vi "write.vi"() -> ()   [LabVIEW 2016]
uses:
  <vilib>/Instr/_visa.llb/VISA Configure Serial Port (Serial Instr).vi
panel:
  in  "Numeric":dbl
  out "Red":bool
  out "yellow":bool
  out "Unit":string
  out "Unit":string
  out "Battery status":bool
  out "Gauge battery Voltage":dbl
  in  "Enable light control":bool
  in  "voltage read length":u32
  out "Voltage feedback":string
  in  "Read":bool
  in  "Cancel Zero reading":bool
  in  "Zero Reading":bool
  in  "Gauge light":bool
  out "Helium underpressure":bool
  out "Numeric 2":dbl
  in  "Set Relay voltage":dbl(slide)=9.0 scale=0.0..10.0
  out "Compressor Status":bool
  in  "Pressure Lower Limit":dbl=0.1
  out "Helium Overpressure":bool
  in  "Pressure Upper Limit":dbl=2.8
  in  "Reading 2":string(combo)="255:R:OTEMP"
  out "Monitor 2":dbl(graph)
  out "Temperature":dbl=23.05
  in  "monitor 2 read length":u32=25
  out "monitor 2 feedback":string
  in  "Reading 1":string(combo)="255:R:MRMD"
  in  "Abort monitoring":bool
  out "Puressure":dbl=0.009
  in  "monitor 1 read length":u32=25
  out "Monitor 1":dbl(graph)
  out "Monitor 1 feedback":string
  # "Gauge Operation"
  # "Relay Configuration"
  # "Serial Port I/O control"
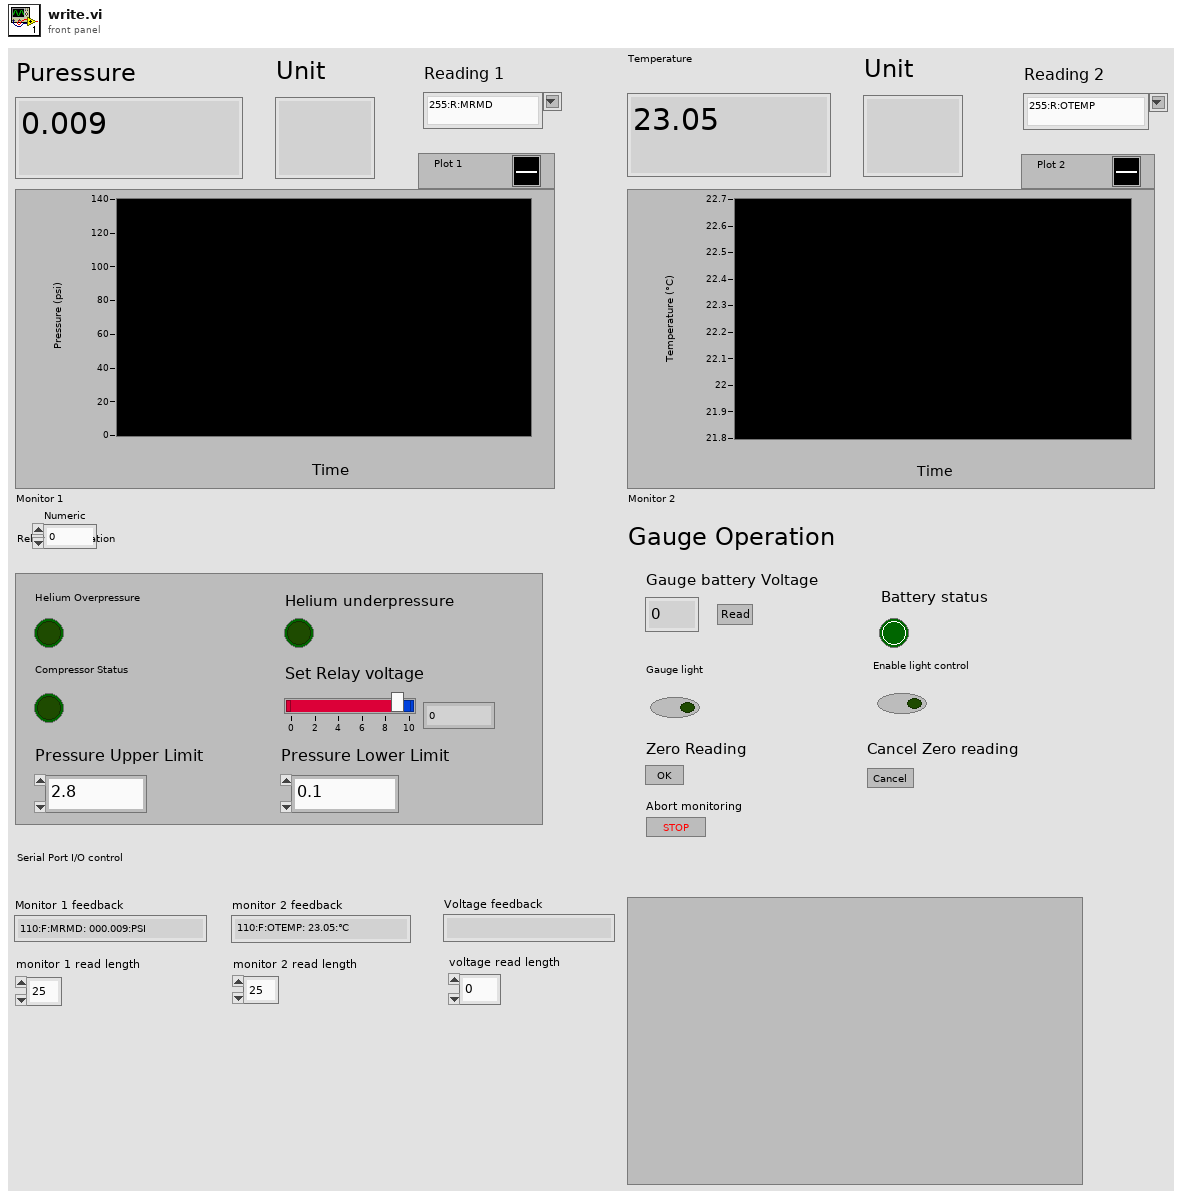
[diagram p1: front panel]
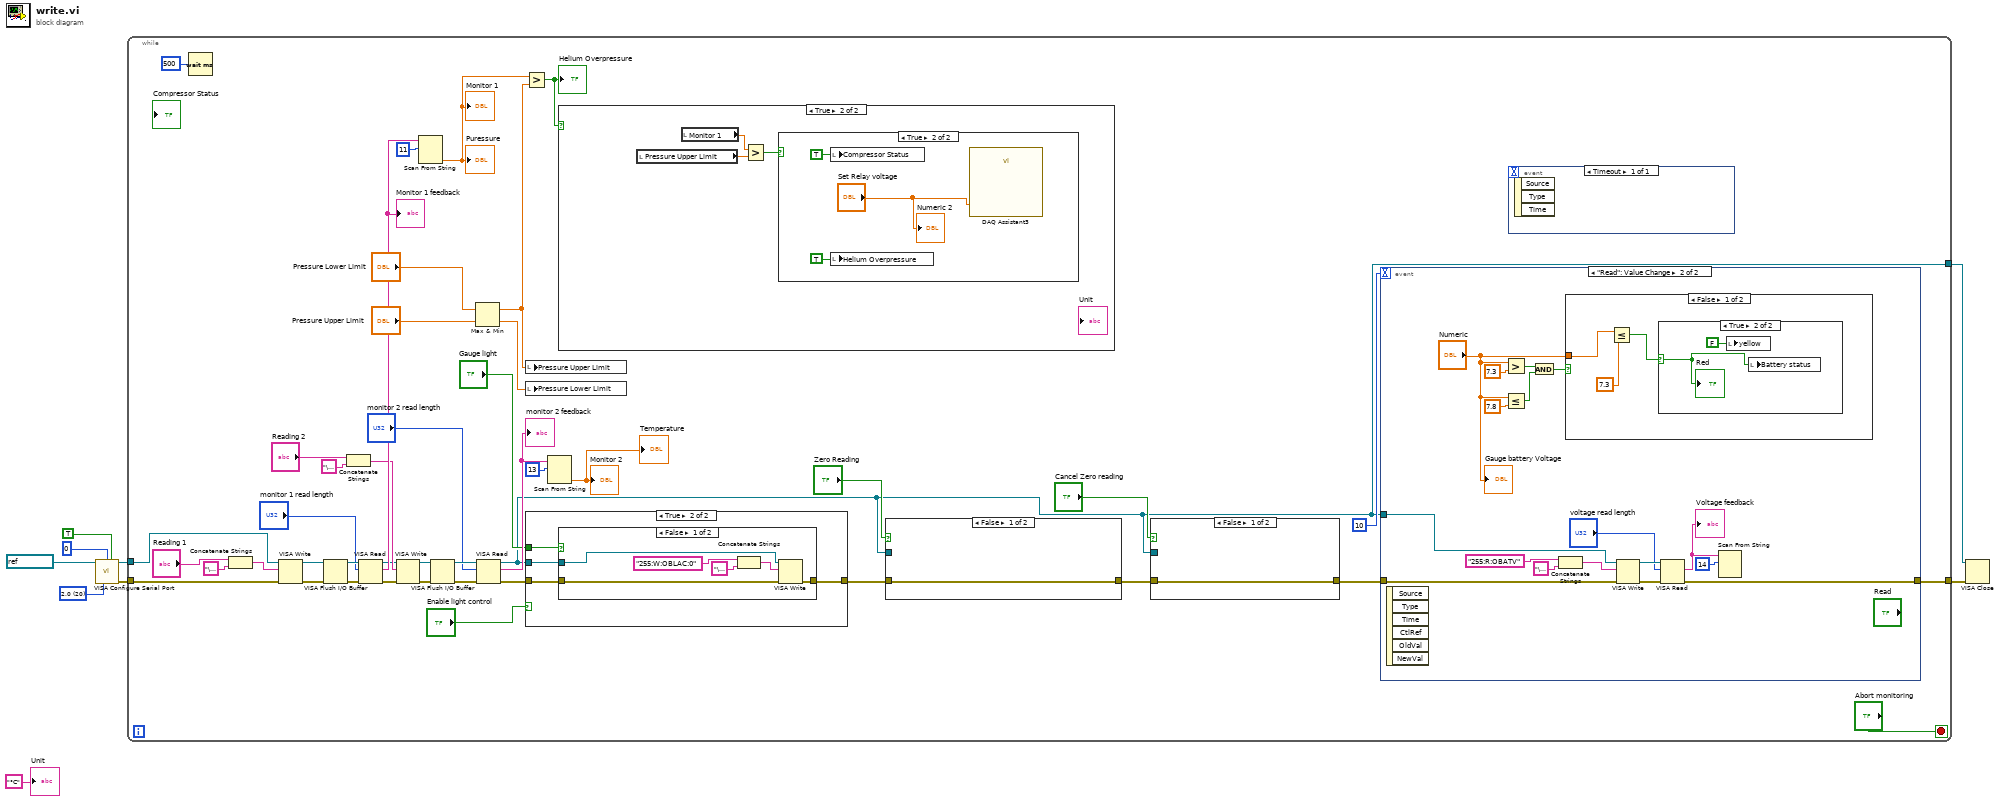
[diagram p0: block diagram]
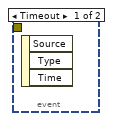
[diagram p2: hidden frame]
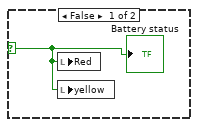
[diagram p3: hidden frame]
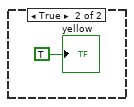
[diagram p4: hidden frame]
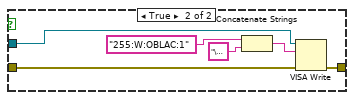
[diagram p6: hidden frame]
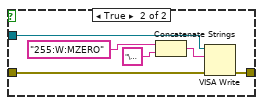
[diagram p7: hidden frame]
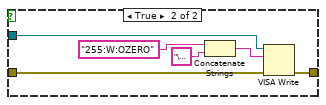
[diagram p8: hidden frame]
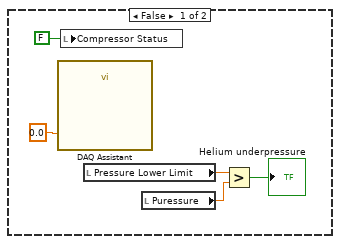
[diagram p9: hidden frame]
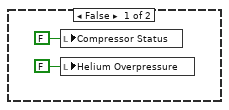
[diagram p10: hidden frame]
diagram:
  w6 = u16 20 items=["1.0"=10, "1.5"=15, "2.0"=20] ("stop bits (10: 1 bit)")
  n1 = call-poly "VISA Configure Serial Port"("VISA resource name"=refnum<visa-resource-name> "COM2", "termination char\n(0xA = '\\n' = LF)"=u8 0 ("termination char\n(0xA = '\\n' = LF)"), "Enable Termination\nChar (T)"=TRUE ("Enable Termination\nChar (T)"), "stop bits (10: 1 bit)"=w6) -> ("VISA resource name out"=w4:refnum<visa-resource-name>, "error out"=w5:errorcluster)  [unwired: 10 in]
  n2 = while {
    tunnel: [w12] -> w3
    tunnel: w5 -> [w45]
    tunnel: w4 -> [w24]
    tunnel: [w10] -> w2
    stop <- "Abort monitoring" stop-if-true
    n3 = Wait (ms)(milliseconds to wait=u32 500) -> ()  [unwired: 1 out]
    n4 = Concatenate Strings("Reading 1", "\u0000") -> (w53:string)
    n5 = VISA Write(VISA resource name=w24, write buffer=w53, error in (no error)=w45) -> (VISA resource name out=w49:refnum<visa-resource-name>, error out=w51:errorcluster)  [unwired: 1 out]
    n6 = VISA Flush I/O Buffer(VISA resource name=w49, error in (no error)=w51) -> (VISA resource name out=w50:refnum<visa-resource-name>, error out=w44:errorcluster)  [unwired: 1 in]
    n7 = Concatenate Strings("Reading 2", "\u0000") -> (w40:string)
    n8 = VISA Read(VISA resource name=w50, byte count="monitor 1 read length", error in (no error)=w44) -> (VISA resource name out=w30:refnum<visa-resource-name>, read buffer=w47:string, error out=w29:errorcluster)  [unwired: 1 out]
    "Monitor 1 feedback" <- w47
    n9 = VISA Write(VISA resource name=w30, write buffer=w40, error in (no error)=w29) -> (VISA resource name out=w36:refnum<visa-resource-name>, error out=w38:errorcluster)  [unwired: 1 out]
    n10 = Scan From String(input string=w47, initial scan location=u32 11) -> (output 1=w21:dbl)  [unwired: 3 in, 3 out]
    "Puressure" <- w21
    "Monitor 1" <- w21
    n11 = VISA Flush I/O Buffer(VISA resource name=w36, error in (no error)=w38) -> (VISA resource name out=w37:refnum<visa-resource-name>, error out=w32:errorcluster)  [unwired: 1 in]
    n12 = Max & Min(x="Pressure Lower Limit", y="Pressure Upper Limit") -> (max(x,y)=w26:dbl, min(x,y)=w25:dbl)
    n13 = VISA Read(VISA resource name=w37, byte count="monitor 2 read length", error in (no error)=w32) -> (VISA resource name out=w12:refnum<visa-resource-name>, read buffer=w34:string, error out=w18:errorcluster)  [unwired: 1 out]
    "monitor 2 feedback" <- w34
    n14 = Greater?(x=w21, y=w26) -> (0:w22:bool)
    "Helium Overpressure" <- w22
    n15 = local write "Pressure Upper Limit"(w26) -> ()
    n16 = local write "Pressure Lower Limit"(w25) -> ()
    n17 = case shown="True" "Enable light control" {
      tunnel: "Gauge light" -> [_ w82]
      tunnel: w18 -> [w78 w81]
      tunnel: [w78 w80] -> w17
      tunnel: w12 -> [_ w79]
      frame False {
      }
      frame True {
        n18 = case shown="False" w82 {
          tunnel: w79 -> [w85 w94]
          tunnel: [w84 w90] -> w80
          tunnel: w81 -> [w83 w89]
          frame False {
            n19 = Concatenate Strings("255:W:OBLAC:0" ("string"), "\u0000" ("string")) -> (w86:string)
            n20 = VISA Write(VISA resource name=w85, write buffer=w86, error in (no error)=w83) -> (error out=w84:errorcluster)  [unwired: 2 out]
          }
          frame True {
            n21 = Concatenate Strings("255:W:OBLAC:1" ("string"), "\u0000" ("string")) -> (w91:string)
            n22 = VISA Write(VISA resource name=w94, write buffer=w91, error in (no error)=w89) -> (error out=w90:errorcluster)  [unwired: 2 out]
          }
        }
      }
    }
    n23 = Scan From String(input string=w34, initial scan location=u32 13) -> (output 1=→"Temperature" →"Monitor 2":dbl)  [unwired: 3 in, 3 out]
    n24 = case shown="True" w22 {
      frame False {
        n25 = call "DAQ Assistant"("data"=0.0) -> ()  [unwired: 17 in, 2 out]
        n26 = local write "Compressor Status"(FALSE ("Compressor Status")) -> ()
        n27 = local read "Pressure Lower Limit"() -> (w113:dbl)
        n28 = local read "Puressure"() -> (w112:dbl)
        n29 = Greater?(x=w113, y=w112) -> (0:→"Helium underpressure":bool)
      }
      frame True {
        n30 = local read "Pressure Upper Limit"() -> (w114:dbl)
        n31 = local read "Monitor 1"() -> (w115:dbl)
        n32 = Greater?(x=w115, y=w114) -> (0:w116:bool)
        n33 = case shown="True" w116 {
          frame False {
            n34 = local write "Compressor Status"(FALSE ("Compressor Status")) -> ()
            n35 = local write "Helium Overpressure"(FALSE ("Helium Overpressure")) -> ()
          }
          frame True {
            n36 = local write "Compressor Status"(TRUE ("Compressor Status")) -> ()
            n37 = local write "Helium Overpressure"(TRUE ("Helium Overpressure")) -> ()
            n38 = call "DAQ Assistant3"("data"="Set Relay voltage") -> ()  [unwired: 17 in, 2 out]
            "Numeric 2" <- "Set Relay voltage"
          }
        }
      }
    }
    n39 = case shown="False" "Zero Reading" {
      tunnel: w12 -> [_ w103]
      tunnel: w17 -> [w102 w105]
      tunnel: [w102 w104] -> w16
      frame False {
      }
      frame True {
        n40 = Concatenate Strings("255:W:OZERO" ("string"), "\u0000" ("string")) -> (w106:string)
        n41 = VISA Write(VISA resource name=w103, write buffer=w106, error in (no error)=w105) -> (error out=w104:errorcluster)  [unwired: 2 out]
      }
    }
    n42 = case shown="False" "Cancel Zero reading" {
      tunnel: w16 -> [w95 w98]
      tunnel: [w95 w97] -> w11
      tunnel: w12 -> [_ w96]
      frame False {
      }
      frame True {
        n43 = Concatenate Strings("255:W:MZERO" ("string"), "\u0000" ("string")) -> (w99:string)
        n44 = VISA Write(VISA resource name=w96, write buffer=w99, error in (no error)=w98) -> (error out=w97:errorcluster)  [unwired: 2 out]
      }
    }
    n45 = event shown="[1] \"Read\": Value Change" {
      selector: _ -> [_ _]
      dyn-events: _ -> [_ _]
      timeout: 10 -> [_ _]
      tunnel: w12 -> [_ w62]
      tunnel: w11 -> [_ w61]
      tunnel: [_ w60] -> w10
      event Timeout {
        n46 = event-data() -> ()  [unwired: 1 in, 3 out]
      }
      event "Read": Value Change {
        n47 = event-data() -> ()  [unwired: 1 in, 6 out]
        n48 = Greater?(x="Numeric", y=7.3) -> (0:w58:bool)
        n49 = Less Or Equal?(x="Numeric", y=7.8) -> (x <= y?=w56:bool)
        n50 = And(x=w58, y=w56) -> (x .and. y?=w55:bool)
        n51 = Concatenate Strings("255:R:OBATV" ("string"), "\u0000" ("string")) -> (w68:string)
        n52 = case shown="False" w55 {
          tunnel: "Numeric" -> [w73 _]
          frame False {
            n53 = Less Or Equal?(x=w73, y=7.3) -> (x <= y?=w71:bool)
            n54 = case shown="True" w71 {
              selector: w71 -> [w74 w75]
              frame False {
                n55 = local write "Red"(w74) -> ()
                n56 = local write "yellow"(w74) -> ()
                "Battery status" <- w74
              }
              frame True {
                n57 = local write "yellow"(FALSE) -> ()
                n58 = local write "Battery status"(w75) -> ()
                "Red" <- w75
              }
            }
          }
          frame True {
            "yellow" <- TRUE
          }
        }
        n59 = VISA Write(VISA resource name=w62, write buffer=w68, error in (no error)=w61) -> (VISA resource name out=w66:refnum<visa-resource-name>, error out=w67:errorcluster)  [unwired: 1 out]
        n60 = VISA Read(VISA resource name=w66, byte count="voltage read length", error in (no error)=w67) -> (read buffer=w64:string, error out=w60:errorcluster)  [unwired: 2 out]
        "Voltage feedback" <- w64
        n61 = Scan From String(input string=w64, initial scan location=u32 14) -> ()  [unwired: 4 in, 3 out]
        "Gauge battery Voltage" <- "Numeric"
      }
    }
    n62 = event shown="[0] Timeout" {
      selector: _ -> [_]
      dyn-events: _ -> [_]
      timeout: _ -> [_]
      event Timeout {
        n63 = event-data() -> ()  [unwired: 1 in, 3 out]
      }
    }
  }
  n64 = VISA Close(VISA resource name=w3, error in (no error)=w2) -> ()  [unwired: 1 out]
  "Unit" <- "°C" ("Unit")
